vi "host.vi"() -> ()   [LabVIEW 2018]
uses:
  <vilib>/userdefined/High Color/nirio_resource_hc.ctl
  <instrlib>/niDCPower/nidcpower.llb/niDCPower Measurement Type.ctl
  <vilib>/FPGAPlugInAG/PXI-7953R/niLvFpga_Open_PXI-7953R.vi
  <vilib>/rvi/interface/common/dynamic/niFpgaDynamicAddResources.vi
  <vilib>/FPGAPlugInAG/Dynamic/niLvFpga_Reset_Dynamic.vi
  <vilib>/FPGAPlugInAG/Dynamic/niLvFpga_Run_Dynamic.vi
  <vilib>/Utility/error.llb/Error Cluster From Error Code.vi
  <vilib>/rvi/errors/niLvFpgaAdjustHostInterfaceError.vi
  <vilib>/FPGAPlugInAG/Dynamic/niLvFpga_Close_Dynamic.vi
  <vilib>/rvi/interface/nirviOpenFPGA/nirviOpenFPGA.xnode
  FPGA Bitfiles/Matrix_Readtarget_Matrixdisplaytar_bV0EX+krGtY.lvbitx
  <vilib>/rvi/interface/nirviMethod/nirviMethod.xnode
  <vilib>/rvi/interface/nirviReadWriteControl/nirviReadWriteControl.xnode
  <vilib>/rvi/interface/nirviCloseFPGA/nirviCloseFPGA.xnode
  <vilib>/FPGAPlugInAG/Dynamic/niLvFpga_ReadFifo_Dynamic.vi
  <vilib>/rvi/errors/niLvFpgaMergeErrorWithErrorCode.vi
  <vilib>/rvi/interface/Simulation/niFpgaSimulationCallBeginRW.vi
  NiFpgaLv.dll
  <vilib>/vision/NI_Vision_Development_Module.lvlib
panel:
  in  "WRITE\nSEL_LOG":bool caption="SEL LOGS"
  out "SEL_log file":refnum<file>
  out "IS_SEL":bool
  in  "SIM_SEL":bool
  in  "VDDIO_limit, mA":dbl=500.0 format="%#_13g"
  in  "VAA_limit, mA":dbl=500.0 format="%#_13g"
  out "selNumVAA":i32 caption="selNum"
  out "selNumVDDIO":i32 caption="selNum"
  in  "voltage level VAA":dbl=5.0 format="%#_13g"
  in  "voltage level VDD":dbl=5.0 format="%#_13g"
  in  "current limit VAA":dbl=0.10000000000000009 format="%#_13g"
  in  "current limit VDD":dbl=0.2 format="%#_13g"
  in  "SEL":path=path "C:/VPL/LabView_PRJ/ПЕЛЕНГ_CMV4000/LOGS/SEL"
  out "Температура":string="25"
  out "Номер образца":string="100"
  out "VDDIO_Current, mA":dbl=-0.21907641736144773 caption="mA" format="%_5g"
  out "VDDIO_Voltage, V":dbl=5.000150980306561 caption="V" format="%_4g"
  out "VAA_Current, mA":dbl=-0.24662982243963988 caption="mA" format="%_5g"
  out "VAA_Voltage, V":dbl=5.000666430855003 caption="V" format="%_4g"
  in  "VAA - VAAPIX":refnum<k15>="PXI1Slot3"
  in  "SEL_time":u32=100
  out "Read_Up":u8 format="%x"
  out "Read_Low":u8=255 format="%x"
  in  "58_ReadData":i16=58
  in  "93_ReadData":i16=93
  out "TIRISTOR":bool
  in  "/RESET":bool=TRUE
  in  "DataLow":u8=231 format="%x"
  in  "Reg":u8=244 format="%x"
  in  "DataUp":u8=2 format="%x"
  in  "Device":u8=186 format="%x"
  in  "VDD_limit, mA":dbl=500.0 format="%#_13g"
  out "selNumVDD":i32 caption="selNum"
  out "Ready":bool=TRUE
  in  "output enabled":bool=TRUE
  out "VDD_Current, mA":dbl=37.395912233375 caption="mA" format="%_5g"
  out "VDD_Voltage, V":dbl=5.000049671830888 caption="V" format="%_4g"
  in  "VDDIO - VDD":refnum<k15>="PXI1Slot2"
  in  "Comand":enum16{"From Controls", "250x250", "RGB565"}(ring)
  in  "Height_pix":i32=250
  in  "Width_pix":i32=250
  in  "55":i16=55
  in  "73":i16=73
  in  "75":i16=75
  in  "56":i16=56
  in  "55":i16=55
  in  "Comand":bool
  out "ACK":u8 format="%b"
  out "String_counter":i16=177
  in  "String_number":i16=250
  in  "I2C_Request":bool
  in  "FALSE_LV":bool
  in  "FALSE_PIXCLK":bool=TRUE
  in  "TRUE_FV":bool=TRUE
  in  "1_EXTCLK_divider":i16=5
  out "Image":T1(plugin-control)
  in  "0_WE divider":i32=3
  in  "50_Rise/Fall divider":i32=50
  in  "72":i16=72
  in  "18":i16=18
  in  "36":i16=36
  in  "54":i16=54
  in  "71":i16=71
  in  "17":i16=17
  in  "35":i16=35
  in  "53":i16=53
  in  "75_Stop":i16=75
  in  "100_Sclk_divider":i32=100
  in  "94":i16=94
  in  "Read1":u8 format="%x"
  in  "Read2":u8 format="%x"
  in  "I2C_Write":bool
  in  "stop":bool
  out "ArrayUp":u64=1534
  out "ArrayLow":u64=2298524764643157990
  in  "resource name":T2="PXI1Slot6" caption="RIO Device"
  out "Сколько вначале":u32=125000
  out "Data":u8[](array[numeric])
  # "YCbCr mode"
  # "VDD"
  # "VDDIO"
  # "VAA"
  # "RGB565"
  # "I2C"
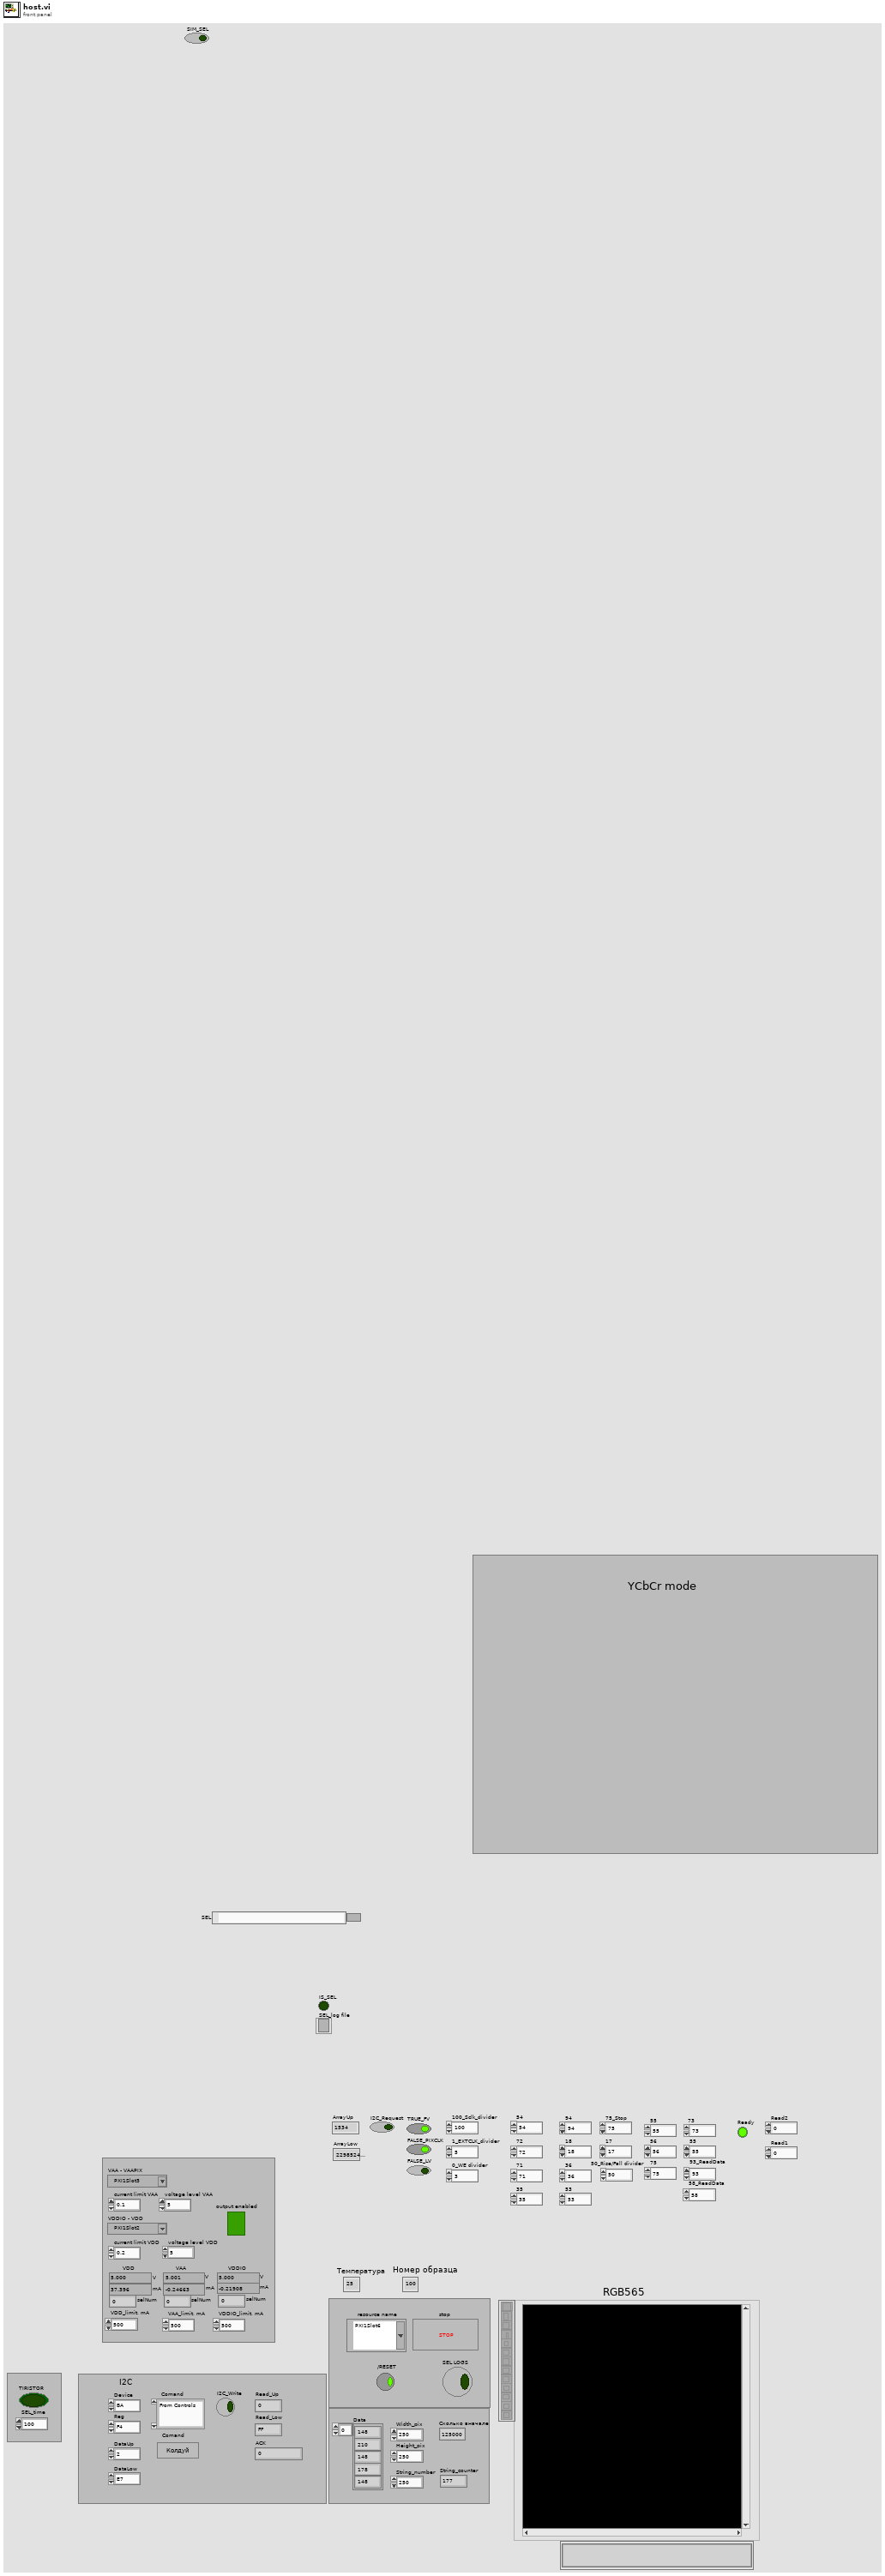
[diagram p1: front panel]
types:
  T1 = typedef "IMAQ Image.ctl" = refnum<image>
  T2 = typedef "nirio_resource_hc.ctl" = tag
  T3 = enum16{"open", "replace", "create", "open or create", "replace or create", "replace or create with confirmation"}
  T4 = typedef "Image Type" = u32
  T5 = typedef "niDCPower Measurement Type.ctl" = i32
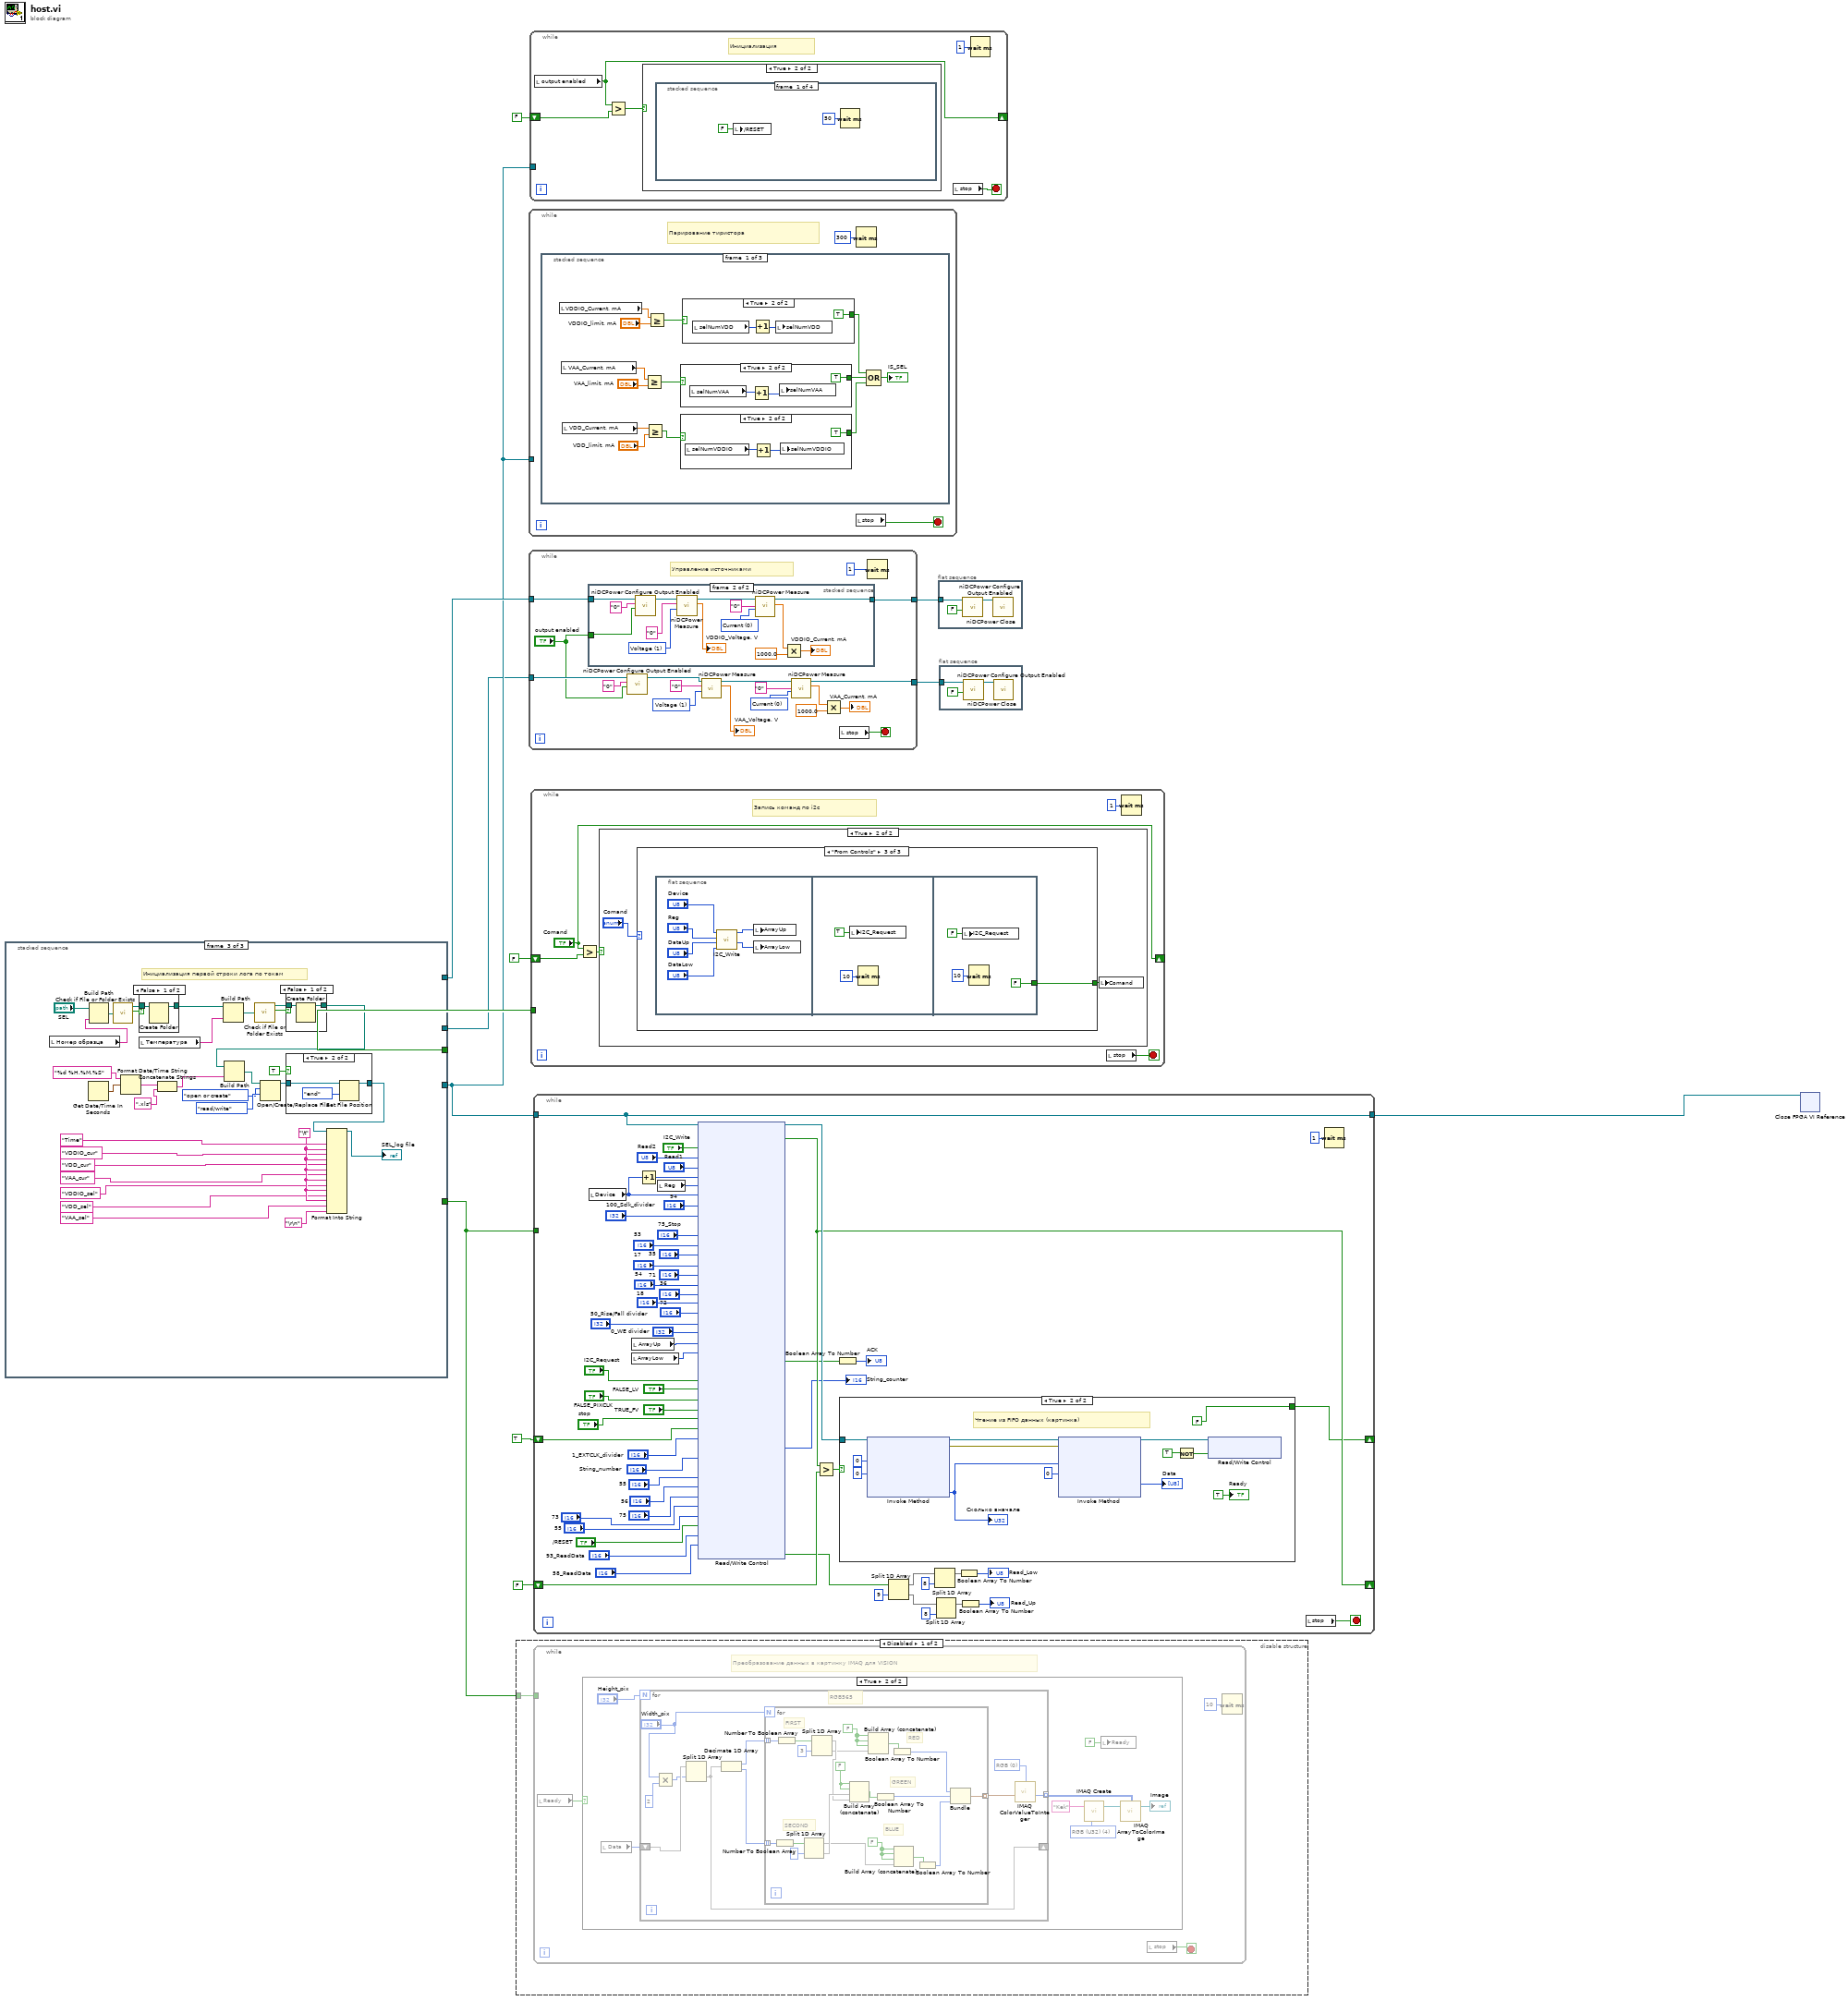
[diagram p0: block diagram]
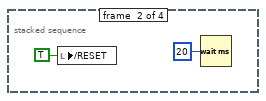
[diagram p5: hidden frame]
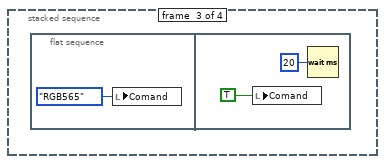
[diagram p6: hidden frame]
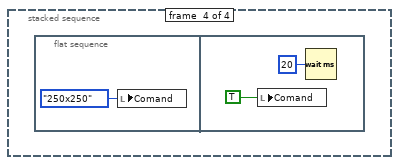
[diagram p7: hidden frame]
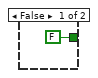
[diagram p8: hidden frame]
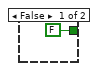
[diagram p9: hidden frame]
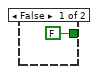
[diagram p10: hidden frame]
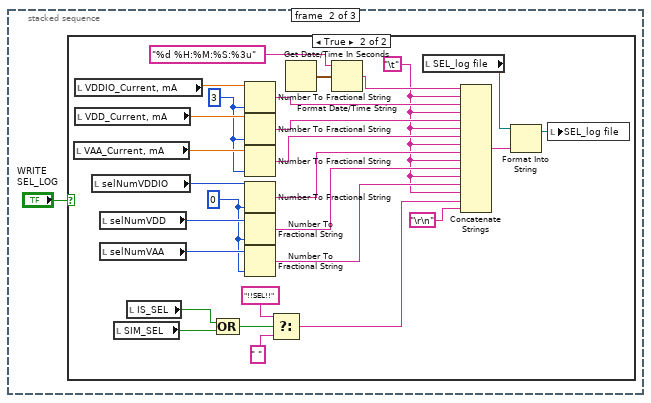
[diagram p11: hidden frame]
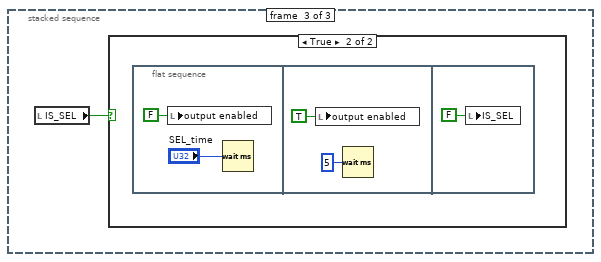
[diagram p13: hidden frame]
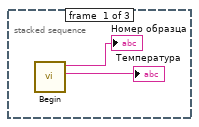
[diagram p15: hidden frame]
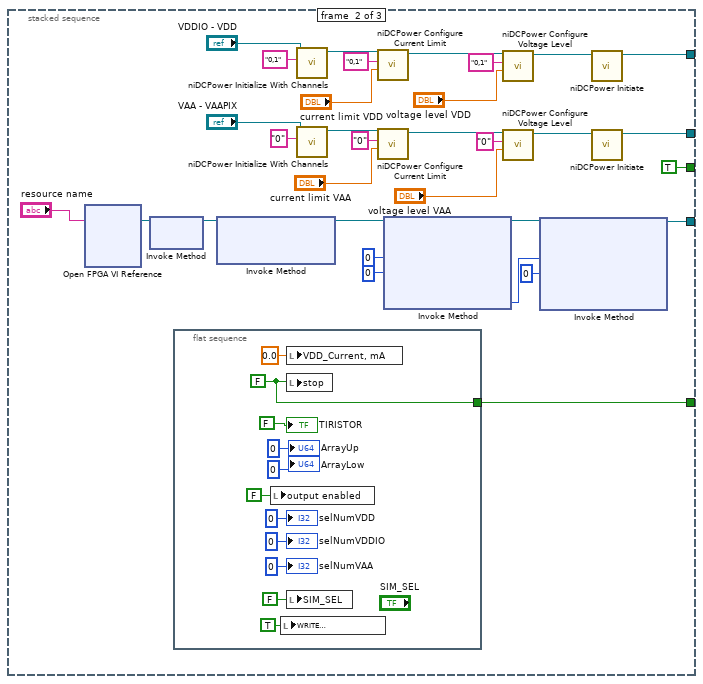
[diagram p16: hidden frame]
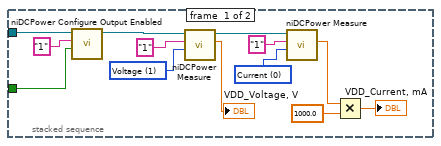
[diagram p20: hidden frame]
diagram:
  n1 = stacked-sequence {
    tunnel: [_ w46 _] -> w3
    tunnel: [_ w27 _] -> w5
    tunnel: [_ w26 _] -> w7
    tunnel: [_ TRUE _] -> w6
    tunnel: [_ w15 _] -> w2
    frame #0 {
      n2 = call "Begin.vi"() -> ("Температура 2"=→"Температура":string, "Номер образца 2"=→"Номер образца":string)  [unwired: 10 in]
    }
    frame #1 {
      n3 = xnode "Open FPGA VI Reference"("resource name"="resource name") -> ("FPGA VI Reference Out"=w36:refnum<k20>)  [unwired: 1 in, 1 out]
      n4 = xnode "Invoke Method"("FPGA VI Reference In"=w36) -> ("FPGA VI Reference Out"=w35:refnum<k20>)  [unwired: 1 in, 1 out]
      n5 = flat-sequence {
        tunnel: [w57] -> w27
        frame #0 {
          w57 = FALSE ("СТОП ПЛИС")
          n6 = local write "output enabled"(FALSE ("output enabled")) -> ()
          n7 = local write "WRITE\nSEL_LOG"(TRUE ("WRITE\nSEL_LOG")) -> ()
          n8 = local write "VDD_Current, mA"(0.0 ("Ch1_Current, mA")) -> ()
          n9 = local write "stop"(w57) -> ()
          n10 = local write "SIM_SEL"(FALSE ("SIM_SEL")) -> ()
          "ArrayLow" <- u64 0 ("ArrayLow")
          "ArrayUp" <- u64 0 ("ArrayUp")
          "selNumVDD" <- 0 ("Numeric")
          "TIRISTOR" <- FALSE ("TIRISTOR")
          "selNumVDDIO" <- 0 ("Numeric")
          "selNumVAA" <- 0 ("Numeric")
        }
      }
      n11 = xnode "Invoke Method"("FPGA VI Reference In"=w35) -> ("FPGA VI Reference Out"=w33:refnum<k20>)  [unwired: 2 in, 1 out]
      n12 = call <instrlib>:"niDCPower Initialize With Channels.vi"("channels"="0,1", "resource name"="VDDIO - VDD") -> ("instrument handle out"=w37:refnum<k15>)  [unwired: 8 in, 1 out]
      n13 = call <instrlib>:"niDCPower Initialize With Channels.vi"("channels"="0", "resource name"="VAA - VAAPIX") -> ("instrument handle out"=w16:refnum<k15>)  [unwired: 8 in, 1 out]
      n14 = call <instrlib>:"niDCPower Configure Current Limit.vi"("current limit"="current limit VDD", "channel name"="0,1", "instrument handle"=w37) -> ("instrument handle out"=w38:refnum<k15>)  [unwired: 7 in, 1 out]
      n15 = call <instrlib>:"niDCPower Configure Current Limit.vi"("current limit"="current limit VAA", "channel name"="0", "instrument handle"=w16) -> ("instrument handle out"=w17:refnum<k15>)  [unwired: 7 in, 1 out]
      n16 = xnode "Invoke Method"("FPGA VI Reference In"=w33, "Number of Elements"=u32 0, "Timeout (ms)"=0) -> ("FPGA VI Reference Out"=w31:refnum<k20>, "Elements Remaining"=w32:u32)  [unwired: 1 in, 2 out]
      n17 = call <instrlib>:"niDCPower Configure Voltage Level.vi"("voltage level"="voltage level VDD", "channel name"="0,1", "instrument handle"=w38) -> ("instrument handle out"=w39:refnum<k15>)  [unwired: 7 in, 1 out]
      n18 = call <instrlib>:"niDCPower Configure Voltage Level.vi"("voltage level"="voltage level VAA", "channel name"="0", "instrument handle"=w17) -> ("instrument handle out"=w18:refnum<k15>)  [unwired: 7 in, 1 out]
      n19 = xnode "Invoke Method"("FPGA VI Reference In"=w31, "Number of Elements"=w32, "Timeout (ms)"=0) -> ("FPGA VI Reference Out"=w46:refnum<k20>)  [unwired: 1 in, 3 out]
      n20 = call <instrlib>:"niDCPower Initiate.vi"("instrument handle"=w39) -> ("instrument handle out"=w26:refnum<k15>)  [unwired: 9 in, 1 out]
      n21 = call <instrlib>:"niDCPower Initiate.vi"("instrument handle"=w18) -> ("instrument handle out"=w15:refnum<k15>)  [unwired: 9 in, 1 out]
    }
    frame #2 {
      w66 = "\t"
      # "Инициализация первой строки лога по токам"
      n22 = local read "Номер образца"() -> (w77:string)
      n23 = Get Date/Time In Seconds() -> (seconds since 1Jan1904=w82:timestamp)
      n24 = Build Path(base path="SEL", name or relative path=w77) -> (appended path=w75:path)
      n25 = call <vilib>:"Check if File or Folder Exists.vi"("path"=w75) -> ("file or folder exists?"=w74:bool, "dup path"=w73:path)  [unwired: 8 in, 1 out]
      n26 = Format Date/Time String(time format string (%c)="%d %H.%M.%S", seconds (now)=w82) -> (date/time string=w84:string)  [unwired: 1 in]
      n27 = case shown="False" w74 {
        tunnel: w73 -> [w98 w99]
        tunnel: [w97 w99] -> w79
        frame False {
          n28 = Create Folder(path (use dialog)=w98) -> (created path=w97:path)  [unwired: 2 in, 2 out]
        }
        frame True {
        }
      }
      n29 = local read "Температура"() -> (w80:string)
      n30 = Concatenate Strings(w84, ".xls" ("string")) -> (w85:string)
      n31 = Build Path(base path=w79, name or relative path=w80) -> (appended path=w88:path)
      n32 = call <vilib>:"Check if File or Folder Exists.vi"("path"=w88) -> ("file or folder exists?"=w89:bool, "dup path"=w78:path)  [unwired: 8 in, 1 out]
      n33 = case shown="False" w89 {
        tunnel: w78 -> [w95 w96]
        tunnel: [w94 w96] -> w86
        frame False {
          n34 = Create Folder(path (use dialog)=w95) -> (created path=w94:path)  [unwired: 2 in, 2 out]
        }
        frame True {
        }
      }
      n35 = Build Path(base path=w86, name or relative path=w85) -> (appended path=w83:path)
      n36 = Open/Create/Replace File(file path (use dialog)=w83, operation (0:open)=T3."open or create", access (0:read/write)=enum16{"read/write", "read-only", "write-only"}."read/write") -> (refnum out=w81:refnum<file>)  [unwired: 3 in, 2 out]
      n37 = case shown="True" TRUE {
        tunnel: w81 -> [w90 w93]
        tunnel: [w90 w91] -> w87
        frame False {
        }
        frame True {
          n38 = Set File Position(refnum=w93, from (0:start)=enum16{"start", "end", "current"}."end") -> (refnum out=w91:refnum<file>)  [unwired: 2 in, 1 out]
        }
      }
      n39 = Format Into String(initial string=w87, "Time" ("input 1"), w66, "VDDIO_cur" ("input 1"), w66, "VDD_cur" ("input 1"), w66, "VAA_cur" ("input 1"), w66, "VDDIO_sel" ("input 1"), w66, "VDD_sel" ("input 1"), w66, "VAA_sel" ("input 1"), "\r\n") -> (resulting string=→"SEL_log file":refnum<file>)  [unwired: 2 in, 1 out]
    }
  }
  n40 = disable-structure shown="Disabled" {
    disable-tunnel: w5 -> [w100 _]
    frame Disabled {
      n41 = while {
        tunnel: w100 -> [_]
        stop <- w103 stop-if-true
        # "Преобразование данных в картинку IMAQ для VISION"
        n42 = local read "Ready"() -> (w101:bool)
        n43 = case shown="True" w101 {
          frame False {
          }
          frame True {
            w110 = T4 4 items=["Grayscale (U8)", "Grayscale (I16)", "Grayscale (SGL)", "Complex (CSG)", "RGB (U32)", "HSL (U32)", "RGB (U64)"] ("Image Type")
            n44 = local read "Data"() -> (w105:u8[])
            n45 = for {
              N: "Height_pix" -> [_]
              shift-right: [w117] -> _
              shift-left: w105 -> [w114]
              tunnel: [w115] -> w106 mode=indexing
              w119 = u16 0 items=["RGB", "HSL", "HSV", "HSI"] ("Color Mode")
              # "RGB565"
              n46 = Multiply(x="Width_pix", y=2) -> (x*y=w113:i32)
              n47 = Split 1D Array(array=w114, index=w113) -> (second subarray=w117:u8[])  [unwired: 1 out]
              n48 = Decimate 1D Array(w117) -> (w121:u8[], w120:u8[])
              n49 = for {
                N: "Width_pix" -> [_]
                tunnel: w121 -> [w140] mode=indexing
                tunnel: w120 -> [w141] mode=indexing
                tunnel: [w122] -> w116 mode=indexing
                w130 = FALSE
                w131 = FALSE
                w132 = FALSE
                # "BLUE"
                # "GREEN"
                # "RED"
                # "SECOND"
                # "FIRST"
                n50 = Number To Boolean Array(number=w141) -> (Boolean array=w136:bool[])
                n51 = Number To Boolean Array(number=w140) -> (Boolean array=w139:bool[])
                n52 = Split 1D Array(array=w136, index=5) -> (first subarray=w128:bool[], second subarray=w135:bool[])
                n53 = Split 1D Array(array=w139, index=3) -> (first subarray=w127:bool[], second subarray=w126:bool[])
                n54 = Build Array (concatenate)(w131, w131, w135, w127) -> (w134:bool[])
                n55 = Build Array (concatenate)(w132, w132, w132, w126) -> (w133:bool[])
                n56 = Boolean Array To Number(Boolean array=w134) -> (number=w124:u8)
                n57 = Boolean Array To Number(Boolean array=w133) -> (number=w123:u8)
                n58 = Build Array (concatenate)(w130, w130, w130, w128) -> (w129:bool[])
                n59 = Boolean Array To Number(Boolean array=w129) -> (number=w125:u8)
                n60 = Bundle(w123, w124, w125) -> (w122:cluster{u8, u8, u8})  [unwired: 1 in]
              }
              n61 = call "IMAQ ColorValueToInteger"("1D Color value array"=w116, "Color Mode"=w119) -> ("1D U32 array"=w115:u32[])  [unwired: 3 in, 3 out]
            }
            n62 = call "IMAQ Create"("Image Name"="Kek", "Image Type"=w110) -> ("New Image"=w109:T1)  [unwired: 3 in, 1 out]
            n63 = local write "Ready"(FALSE ("Ready")) -> ()
            n64 = call "IMAQ ArrayToColorImage"("Image Pixels (U32)"=w106, "Image"=w109) -> ("Image Out"=→"Image":T1)  [unwired: 3 in, 1 out]
          }
        }
        n65 = local read "stop"() -> (w103:bool)
        n66 = Wait (ms)(milliseconds to wait=u32 10) -> ()  [unwired: 1 out]
      }
    }
    frame Enabled {
    }
  }
  n67 = while {
    tunnel: w3 -> [_]
    stop <- w143 stop-if-true
    # "Парирование тиристора"
    n68 = stacked-sequence {
      frame #0 {
        n69 = local read "VDDIO_Current, mA"() -> (w151:dbl)
        n70 = local read "VAA_Current, mA"() -> (w152:dbl)
        n71 = local read "VDD_Current, mA"() -> (w156:dbl)
        n72 = Greater Or Equal?(x=w152, y="VAA_limit, mA") -> (x >= y?=w148:bool)
        n73 = Greater Or Equal?(x=w156, y="VDD_limit, mA") -> (x >= y?=w146:bool)
        n74 = Greater Or Equal?(x=w151, y="VDDIO_limit, mA") -> (x >= y?=w150:bool)
        n75 = case shown="True" w148 {
          tunnel: [FALSE TRUE] -> w147
          frame False {
          }
          frame True {
            n76 = local read "selNumVAA"() -> (w164:i32)
            n77 = Increment(x=w164) -> (x+1=w163:i32)
            n78 = local write "selNumVAA"(w163) -> ()
          }
        }
        n79 = case shown="True" w146 {
          tunnel: [FALSE TRUE] -> w145
          frame False {
          }
          frame True {
            n80 = local read "selNumVDDIO"() -> (w160:i32)
            n81 = Increment(x=w160) -> (x+1=w159:i32)
            n82 = local write "selNumVDDIO"(w159) -> ()
          }
        }
        n83 = case shown="True" w150 {
          tunnel: [FALSE TRUE] -> w149
          frame False {
          }
          frame True {
            n84 = local read "selNumVDD"() -> (w168:i32)
            n85 = Increment(x=w168) -> (x+1=w167:i32)
            n86 = local write "selNumVDD"(w167) -> ()
          }
        }
        n87 = Compound Arithmetic op=OR(w149, w147, w145) -> (→"IS_SEL":bool)
      }
      frame #1 {
        n88 = case shown="True" "WRITE\nSEL_LOG" {
          frame False {
          }
          frame True {
            w176 = i16 0 ("width (-)")
            w175 = i16 3 ("width (-)")
            w173 = "\t"
            n89 = local read "VAA_Current, mA"() -> (w190:dbl)
            n90 = local read "VDDIO_Current, mA"() -> (w188:dbl)
            n91 = local read "VDD_Current, mA"() -> (w189:dbl)
            n92 = local read "selNumVDDIO"() -> (w191:i32)
            n93 = local read "selNumVDD"() -> (w192:i32)
            n94 = local read "selNumVAA"() -> (w193:i32)
            n95 = local read "SIM_SEL"() -> (w180:bool)
            n96 = local read "IS_SEL"() -> (w181:bool)
            n97 = Compound Arithmetic op=OR(w181, w180) -> (w197:bool)
            n98 = Number To Fractional String(number=w188, precision (6)=w175) -> (F-format string=w194:string)  [unwired: 2 in]
            n99 = Number To Fractional String(number=w189, precision (6)=w175) -> (F-format string=w195:string)  [unwired: 2 in]
            n100 = Number To Fractional String(number=w190, precision (6)=w175) -> (F-format string=w196:string)  [unwired: 2 in]
            n101 = Number To Fractional String(number=w191, precision (6)=w176) -> (F-format string=w184:string)  [unwired: 2 in]
            n102 = Number To Fractional String(number=w192, precision (6)=w176) -> (F-format string=w183:string)  [unwired: 2 in]
            n103 = Number To Fractional String(number=w193, precision (6)=w176) -> (F-format string=w182:string)  [unwired: 2 in]
            n104 = Select(t="!!SEL!!", s=w197, f=" ") -> (s? t:f=w179:string)
            n105 = Get Date/Time In Seconds() -> (seconds since 1Jan1904=w185:timestamp)
            n106 = Format Date/Time String(time format string (%c)="%d %H:%M:%S:%3u", seconds (now)=w185) -> (date/time string=w187:string)  [unwired: 1 in]
            n107 = local read "SEL_log file"() -> (w171:refnum<file>)
            n108 = Concatenate Strings(w187, w173, w194, w173, w195, w173, w196, w173, w184, w173, w183, w173, w182, w173, w179, "\r\n") -> (w186:string)
            n109 = Format Into String(initial string=w171, w186) -> (resulting string=w170:refnum<file>)  [unwired: 2 in, 1 out]
            n110 = local write "SEL_log file"(w170) -> ()
          }
        }
      }
      frame #2 {
        n111 = local read "IS_SEL"() -> (w198:bool)
        n112 = case shown="True" w198 {
          frame False {
          }
          frame True {
            n113 = flat-sequence {
              frame #0 {
                n114 = local write "output enabled"(FALSE ("output enabled")) -> ()
                n115 = Wait (ms)(milliseconds to wait="SEL_time") -> ()  [unwired: 1 out]
              }
              frame #1 {
                n116 = local write "output enabled"(TRUE ("output enabled")) -> ()
                n117 = Wait (ms)(milliseconds to wait=u32 5) -> ()  [unwired: 1 out]
              }
              frame #2 {
                n118 = local write "IS_SEL"(FALSE ("IS_SEL")) -> ()
              }
            }
          }
        }
      }
    }
    n119 = local read "stop"() -> (w143:bool)
    n120 = Wait (ms)(milliseconds to wait=u32 300) -> ()  [unwired: 1 out]
  }
  n121 = while {
    tunnel: w7 -> [w220]
    tunnel: [w219] -> w9
    tunnel: w2 -> [w206]
    tunnel: [w207] -> w1
    stop <- w221 stop-if-true
    w210 = T5 0 items=["Current", "Voltage"] ("measurement type")
    w211 = T5 1 items=["Current", "Voltage"] ("measurement type")
    # "Управление источниками"
    n122 = stacked-sequence {
      tunnel: w220 -> [w232 w237]
      tunnel: [_ w236] -> w219
      tunnel: "output enabled" -> [w222 w238]
      frame #0 {
        w225 = T5 0 items=["Current", "Voltage"] ("measurement type")
        w226 = T5 1 items=["Current", "Voltage"] ("measurement type")
        n123 = call <instrlib>:"niDCPower Configure Output Enabled.vi"("output enabled"=w222, "channel name"="1", "instrument handle"=w232) -> ("instrument handle out"=w234:refnum<k15>)  [unwired: 7 in, 1 out]
        n124 = call <instrlib>:"niDCPower Measure.vi"("measurement type"=w226, "channel name"="1", "instrument handle"=w234) -> ("measurement"=→"VDD_Voltage, V":dbl, "instrument handle out"=w231:refnum<k15>)  [unwired: 6 in, 1 out]
        n125 = call <instrlib>:"niDCPower Measure.vi"("measurement type"=w225, "channel name"="1", "instrument handle"=w231) -> ("measurement"=w227:dbl)  [unwired: 6 in, 2 out]
        n126 = Multiply(x=w227, y=1000.0) -> (x*y=→"VDD_Current, mA":dbl)
      }
      frame #1 {
        w243 = T5 0 items=["Current", "Voltage"] ("measurement type")
        w241 = T5 1 items=["Current", "Voltage"] ("measurement type")
        n127 = call <instrlib>:"niDCPower Configure Output Enabled.vi"("output enabled"=w238, "channel name"="0", "instrument handle"=w237) -> ("instrument handle out"=w245:refnum<k15>)  [unwired: 7 in, 1 out]
        n128 = call <instrlib>:"niDCPower Measure.vi"("measurement type"=w241, "channel name"="0", "instrument handle"=w245) -> ("measurement"=→"VDDIO_Voltage, V":dbl, "instrument handle out"=w246:refnum<k15>)  [unwired: 6 in, 1 out]
        n129 = call <instrlib>:"niDCPower Measure.vi"("measurement type"=w243, "channel name"="0", "instrument handle"=w246) -> ("measurement"=w247:dbl, "instrument handle out"=w236:refnum<k15>)  [unwired: 6 in, 1 out]
        n130 = Multiply(x=w247, y=1000.0) -> (x*y=→"VDDIO_Current, mA":dbl)
      }
    }
    n131 = call <instrlib>:"niDCPower Configure Output Enabled.vi"("output enabled"="output enabled", "channel name"="0", "instrument handle"=w206) -> ("instrument handle out"=w218:refnum<k15>)  [unwired: 7 in, 1 out]
    n132 = call <instrlib>:"niDCPower Measure.vi"("measurement type"=w211, "channel name"="0", "instrument handle"=w218) -> ("measurement"=→"VAA_Voltage, V":dbl, "instrument handle out"=w216:refnum<k15>)  [unwired: 6 in, 1 out]
    n133 = call <instrlib>:"niDCPower Measure.vi"("measurement type"=w210, "channel name"="0", "instrument handle"=w216) -> ("measurement"=w212:dbl, "instrument handle out"=w207:refnum<k15>)  [unwired: 6 in, 1 out]
    n134 = Multiply(x=w212, y=1000.0) -> (x*y=→"VAA_Current, mA":dbl)
    n135 = local read "stop"() -> (w221:bool)
    n136 = Wait (ms)(milliseconds to wait=u32 1) -> ()  [unwired: 1 out]
  }
  n137 = while {
    shift-right: [w249] -> _
    shift-left: FALSE -> [w252]
    tunnel: w3 -> [_]
    stop <- w253 stop-if-true
    # "Инициализация"
    n138 = local read "output enabled"() -> (w249:bool)
    n139 = Greater?(x=w249, y=w252) -> (0:w251:bool)
    n140 = case shown="True" w251 {
      frame False {
      }
      frame True {
        n141 = stacked-sequence {
          frame #0 {
            n142 = local write "/RESET"(FALSE ("RESET")) -> ()
            n143 = Wait (ms)(milliseconds to wait=u32 50) -> ()  [unwired: 1 out]
          }
          frame #1 {
            n144 = local write "/RESET"(TRUE ("RESET")) -> ()
            n145 = Wait (ms)(milliseconds to wait=u32 20) -> ()  [unwired: 1 out]
          }
          frame #2 {
            n146 = flat-sequence {
              frame #0 {
                n147 = local write "Comand"(enum16{"From Controls", "250x250", "RGB565"}."RGB565" ("Comand")) -> ()
              }
              frame #1 {
                n148 = local write "Comand"(TRUE) -> ()
                n149 = Wait (ms)(milliseconds to wait=u32 20) -> ()  [unwired: 1 out]
              }
            }
          }
          frame #3 {
            n150 = flat-sequence {
              frame #0 {
                n151 = local write "Comand"(enum16{"From Controls", "250x250", "RGB565"}."250x250" ("Comand")) -> ()
              }
              frame #1 {
                n152 = local write "Comand"(TRUE) -> ()
                n153 = Wait (ms)(milliseconds to wait=u32 20) -> ()  [unwired: 1 out]
              }
            }
          }
        }
      }
    }
    n154 = local read "stop"() -> (w253:bool)
    n155 = Wait (ms)(milliseconds to wait=u32 1) -> ()  [unwired: 1 out]
  }
  n156 = while {
    shift-right: ["Comand"] -> _
    shift-left: FALSE -> [w266]
    tunnel: w6 -> [_]
    stop <- w268 stop-if-true
    # "Запись команд по i2c"
    n157 = Greater?(x="Comand", y=w266) -> (0:w267:bool)
    n158 = case shown="True" w267 {
      frame False {
      }
      frame True {
        n159 = case shown="\"From Controls\"" "Comand" {
          tunnel: [w271 w297 w322] -> w269
          frame "RGB565" {
            n160 = stacked-sequence {
              tunnel: [_ w283] -> w271
              frame #0 {
                n161 = flat-sequence {
                  frame #0 {
                    n162 = local write "I2C_Write"(TRUE ("I2C_Write")) -> ()
                    n163 = call "I2C_Write.vi"("DataLow"=u8 1 ("Device"), "DataUp"=u8 0 ("Device"), "Reg"=u8 240 ("Device"), "Device"=u8 186) -> ("ArrayLow"=w277:u64, "ArrayUp"=w276:u64)  [unwired: 6 in]
                    n164 = local write "ArrayUp"(w276) -> ()
                    n165 = local write "ArrayLow"(w277) -> ()
                  }
                  frame #1 {
                    n166 = local write "I2C_Request"(TRUE ("I2C_Request")) -> ()
                    n167 = Wait (ms)(milliseconds to wait=u32 5) -> ()  [unwired: 1 out]
                  }
                  frame #2 {
                    n168 = local write "I2C_Request"(FALSE ("I2C_Request")) -> ()
                    n169 = Wait (ms)(milliseconds to wait=u32 5) -> ()  [unwired: 1 out]
                  }
                }
              }
              frame #1 {
                n170 = flat-sequence {
                  tunnel: [FALSE ("RGB565")] -> w283
                  frame #0 {
                    n171 = local write "I2C_Write"(TRUE ("I2C_Write")) -> ()
                    n172 = call "I2C_Write.vi"("DataLow"=u8 0 ("Device"), "DataUp"=u8 3 ("Device"), "Reg"=u8 58 ("Device"), "Device"=u8 186) -> ("ArrayLow"=w289:u64, "ArrayUp"=w288:u64)  [unwired: 6 in]
                    n173 = local write "ArrayUp"(w288) -> ()
                    n174 = local write "ArrayLow"(w289) -> ()
                  }
                  frame #1 {
                    n175 = local write "I2C_Request"(TRUE ("I2C_Request")) -> ()
                    n176 = Wait (ms)(milliseconds to wait=u32 2) -> ()  [unwired: 1 out]
                  }
                  frame #2 {
                    n177 = local write "I2C_Request"(FALSE ("I2C_Request")) -> ()
                    n178 = Wait (ms)(milliseconds to wait=u32 2) -> ()  [unwired: 1 out]
                  }
                }
              }
            }
          }
          frame "250x250" {
            w296 = 250 ("Height_pix")
            n179 = stacked-sequence {
              tunnel: [_ w309] -> w297
              frame #0 {
                n180 = flat-sequence {
                  frame #0 {
                    n181 = local write "I2C_Write"(TRUE ("I2C_Write")) -> ()
                    n182 = call "I2C_Write.vi"("DataLow"=u8 0 ("Device"), "DataUp"=u8 0 ("Device"), "Reg"=u8 240 ("Device"), "Device"=u8 186) -> ("ArrayLow"=w303:u64, "ArrayUp"=w302:u64)  [unwired: 6 in]
                    n183 = local write "ArrayUp"(w302) -> ()
                    n184 = local write "ArrayLow"(w303) -> ()
                  }
                  frame #1 {
                    n185 = local write "I2C_Request"(TRUE ("I2C_Request")) -> ()
                    n186 = Wait (ms)(milliseconds to wait=u32 10) -> ()  [unwired: 1 out]
                  }
                  frame #2 {
                    n187 = local write "I2C_Request"(FALSE ("I2C_Request")) -> ()
                    n188 = Wait (ms)(milliseconds to wait=u32 10) -> ()  [unwired: 1 out]
                  }
                }
              }
              frame #1 {
                n189 = flat-sequence {
                  tunnel: [FALSE ("RGB565")] -> w309
                  frame #0 {
                    n190 = local write "I2C_Write"(TRUE ("I2C_Write")) -> ()
                    n191 = call "I2C_Write.vi"("DataLow"=u8 231 ("Device"), "DataUp"=u8 1 ("Device"), "Reg"=u8 4 ("Device"), "Device"=u8 186) -> ("ArrayLow"=w311:u64, "ArrayUp"=w310:u64)  [unwired: 6 in]
                    n192 = local write "ArrayUp"(w310) -> ()
                    n193 = local write "ArrayLow"(w311) -> ()
                  }
                  frame #1 {
                    n194 = local write "I2C_Request"(TRUE ("I2C_Request")) -> ()
                    n195 = Wait (ms)(milliseconds to wait=u32 10) -> ()  [unwired: 1 out]
                  }
                  frame #2 {
                    n196 = local write "I2C_Request"(FALSE ("I2C_Request")) -> ()
                    n197 = Wait (ms)(milliseconds to wait=u32 10) -> ()  [unwired: 1 out]
                  }
                }
              }
            }
            n198 = local write "String_number"(w296) -> ()
            n199 = local write "Width_pix"(w296) -> ()
            n200 = local write "Height_pix"(w296) -> ()
          }
          frame "From Controls" {
            n201 = flat-sequence {
              tunnel: [FALSE] -> w322
              frame #0 {
                n202 = call "I2C_Write.vi"("DataLow"="DataLow", "DataUp"="DataUp", "Reg"="Reg", "Device"="Device") -> ("ArrayLow"=w324:u64, "ArrayUp"=w323:u64)  [unwired: 6 in]
                n203 = local write "ArrayUp"(w323) -> ()
                n204 = local write "ArrayLow"(w324) -> ()
              }
              frame #1 {
                n205 = local write "I2C_Request"(TRUE ("I2C_Request")) -> ()
                n206 = Wait (ms)(milliseconds to wait=u32 10) -> ()  [unwired: 1 out]
              }
              frame #2 {
                n207 = local write "I2C_Request"(FALSE ("I2C_Request")) -> ()
                n208 = Wait (ms)(milliseconds to wait=u32 10) -> ()  [unwired: 1 out]
              }
            }
          }
        }
        n209 = local write "Comand"(w269) -> ()
      }
    }
    n210 = local read "stop"() -> (w268:bool)
    n211 = Wait (ms)(milliseconds to wait=u32 1) -> ()  [unwired: 1 out]
  }
  n212 = while {
    tunnel: w3 -> [w390]
    tunnel: [w390] -> w12
    shift-right: [w371] -> _
    shift-left: FALSE -> [w391]
    tunnel: w5 -> [_]
    shift-right: [w352] -> _
    shift-left: TRUE -> [w353]
    stop <- w351 stop-if-true
    n213 = local read "Device"() -> (w348:u8)
    n214 = local read "ArrayLow"() -> (w365:u64)
    n215 = local read "ArrayUp"() -> (w364:u64)
    n216 = Increment(x=w348) -> (x+1=w347:u8)
    n217 = local read "Reg"() -> (w346:u8)
    n218 = xnode "Read/Write Control"("FPGA VI Reference In"=w390, "I2C_Write"="I2C_Write", "Read2"="Read2", "Read1"="Read1", "Device_Read"=w347, "Reg"=w346, "Device_Write"=w348, "93"="94", "100_Sclk_divider"="100_Sclk_divider", "75_Stop"="75_Stop", "53"="53", "35"="35", "17"="17", "71"="71", "54"="54", "36"="36", "18"="18", "72"="72", "50_Rise/Fall divider"="50_Rise/Fall divider", "0_WE divider"="0_WE divider", "DataUp"=w364, "DataLow"=w365, "I2C_Request"="I2C_Request", "FALSE_LV"="FALSE_LV", "FALSE_PIXCLK"="FALSE_PIXCLK", "TRUE_FV"="TRUE_FV", "Остановите"="stop", "Читай_Линию"=w353, "1_EXTCLK_divider"="1_EXTCLK_divider", "String_number"="String_number", "55"="55", "56"="56", "75"="75", "73"="73", "55"="55", "RESET"="/RESET", "93_ReadData"="93_ReadData", "58_ReadData"="58_ReadData") -> ("FPGA VI Reference Out"=w389:refnum<k20>, "Линия_готова_на_все"=w371:bool, "ACK"=w360:bool[], "String_counter"=→"String_counter":i16, "Array_ReadData"=w343:bool[])  [unwired: 2 in, 3 out]
    n219 = Greater?(x=w371, y=w391) -> (0:w361:bool)
    n220 = Boolean Array To Number(Boolean array=w360) -> (number=→"ACK":u8)
    n221 = case shown="True" w361 {
      tunnel: w389 -> [_ w400]
      tunnel: [TRUE FALSE ("Читай_Линию")] -> w352
      frame False {
      }
      frame True {
        # "Чтение из FIFO данных (картинка)"
        n222 = xnode "Invoke Method"("FPGA VI Reference In"=w400, "Number of Elements"=u32 0, "Timeout (ms)"=0) -> ("FPGA VI Reference Out"=w405:refnum<k20>, "error out"=w404:errorcluster, "Elements Remaining"=w396:u32)  [unwired: 1 in, 1 out]
        "Сколько вначале" <- w396
        n223 = xnode "Invoke Method"("FPGA VI Reference In"=w405, "error in"=w404, "Number of Elements"=w396, "Timeout (ms)"=0) -> ("FPGA VI Reference Out"=w397:refnum<k20>, "Data"=→"Data":u8[])  [unwired: 2 out]
        n224 = Not(x=TRUE) -> (.not. x?=w398:bool)
        n225 = xnode "Read/Write Control"("FPGA VI Reference In"=w397, "Линия_ прочтена"=w398) -> ()  [unwired: 1 in, 2 out]
        "Ready" <- TRUE ("Ready")
      }
    }
    n226 = Split 1D Array(array=w343, index=9) -> (first subarray=w337:bool[], second subarray=w341:bool[])
    n227 = Split 1D Array(array=w337, index=8) -> (first subarray=w336:bool[])  [unwired: 1 out]
    n228 = Split 1D Array(array=w341, index=8) -> (first subarray=w334:bool[])  [unwired: 1 out]
    n229 = Boolean Array To Number(Boolean array=w336) -> (number=→"Read_Low":u8)
    n230 = Boolean Array To Number(Boolean array=w334) -> (number=→"Read_Up":u8)
    n231 = local read "stop"() -> (w351:bool)
    n232 = Wait (ms)(milliseconds to wait=u32 1) -> ()  [unwired: 1 out]
  }
  n233 = flat-sequence {
    tunnel: w9 -> [w408]
    frame #0 {
      n234 = call <instrlib>:"niDCPower Configure Output Enabled.vi"("output enabled"=FALSE, "instrument handle"=w408) -> ("instrument handle out"=w406:refnum<k15>)  [unwired: 8 in, 1 out]
      n235 = call <instrlib>:"niDCPower Close.vi"("instrument handle"=w406) -> ()  [unwired: 10 in, 1 out]
    }
  }
  n236 = flat-sequence {
    tunnel: w1 -> [w411]
    frame #0 {
      n237 = call <instrlib>:"niDCPower Configure Output Enabled.vi"("output enabled"=FALSE, "instrument handle"=w411) -> ("instrument handle out"=w409:refnum<k15>)  [unwired: 8 in, 1 out]
      n238 = call <instrlib>:"niDCPower Close.vi"("instrument handle"=w409) -> ()  [unwired: 10 in, 1 out]
    }
  }
  n239 = xnode "Close FPGA VI Reference"("FPGA VI Reference In"=w12) -> ()  [unwired: 1 in, 1 out]
